vi "Translate to Array Data_BU3.vi"(8 "modified error":errorcluster, 9 "modified data":path=path "C:/Users/User/Desktop/test.csv", 10 "original error":errorcluster, 11 "original data":path=path "C:/Users/User/Desktop/aaa.csv") -> ()   [LabVIEW 2023]
uses:
  <vilib>/Utility/error.llb/DialogType.ctl
panel:
  in  "External\nRef":bool=TRUE
  out "x/y":dbl[](array[numeric])
  in  "Current Mode":u8[][](array[numeric])
  in  "Electrode number, N":u16=8
  out "number 2":i32
  out "number":i32
  in  "Only Use Last Value?":bool=TRUE
  in  "Array Mode":u16(ring) items=["Gradient + Dipole dipole", "Gradient", "Dipole Dipole", "Schlumberger"]
  in  "Insert\nBreak":bool=TRUE
  in  "Inverse\nPolarity":bool=TRUE
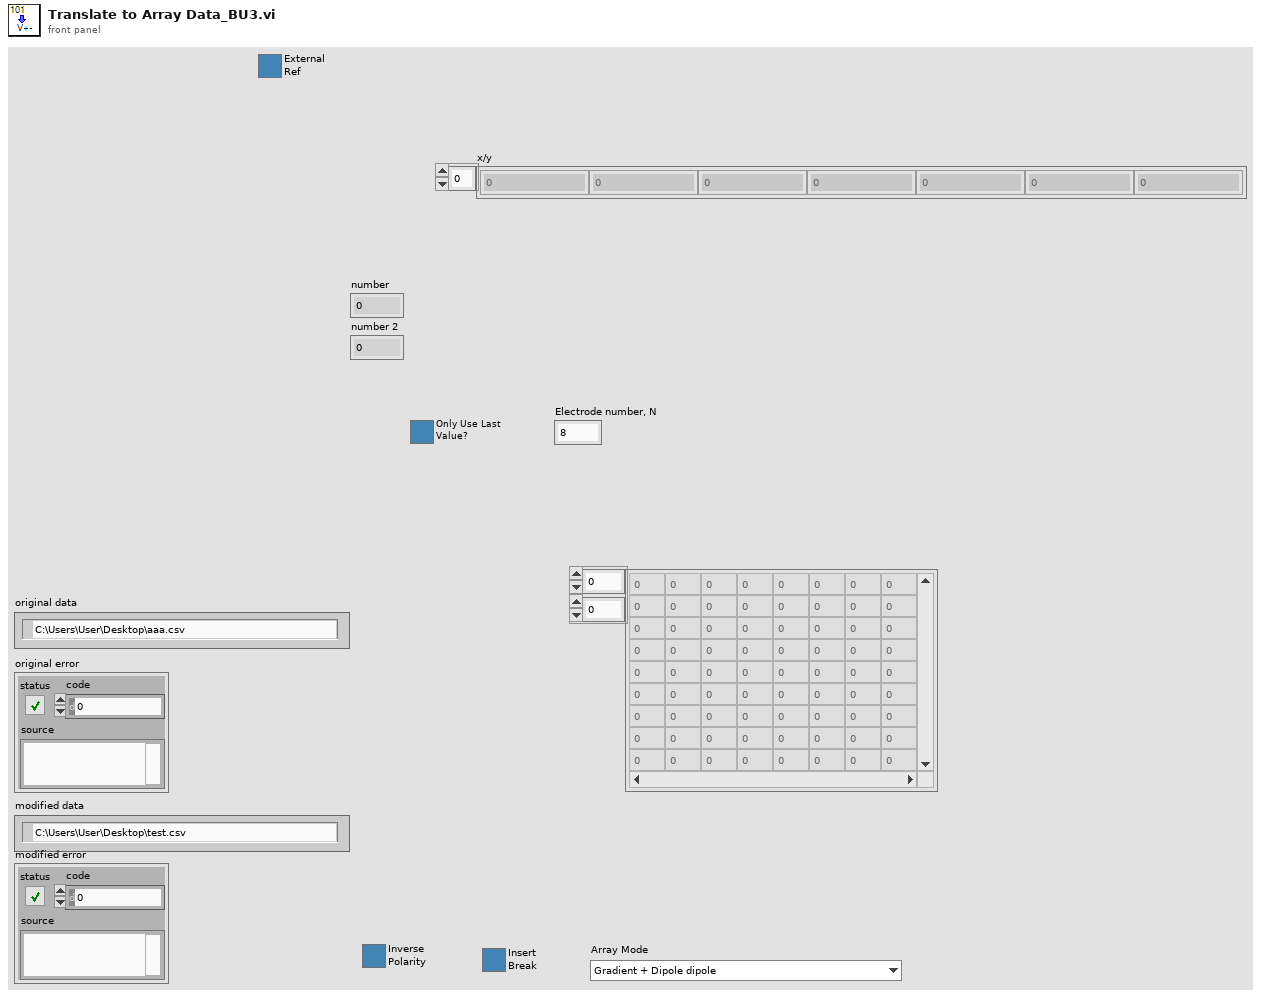
[diagram p1: front panel]
types:
  T1 = enum16{"open", "replace", "create", "open or create", "replace or create", "replace or create with confirmation"}
  T2 = typedef "DialogType.ctl" = u16
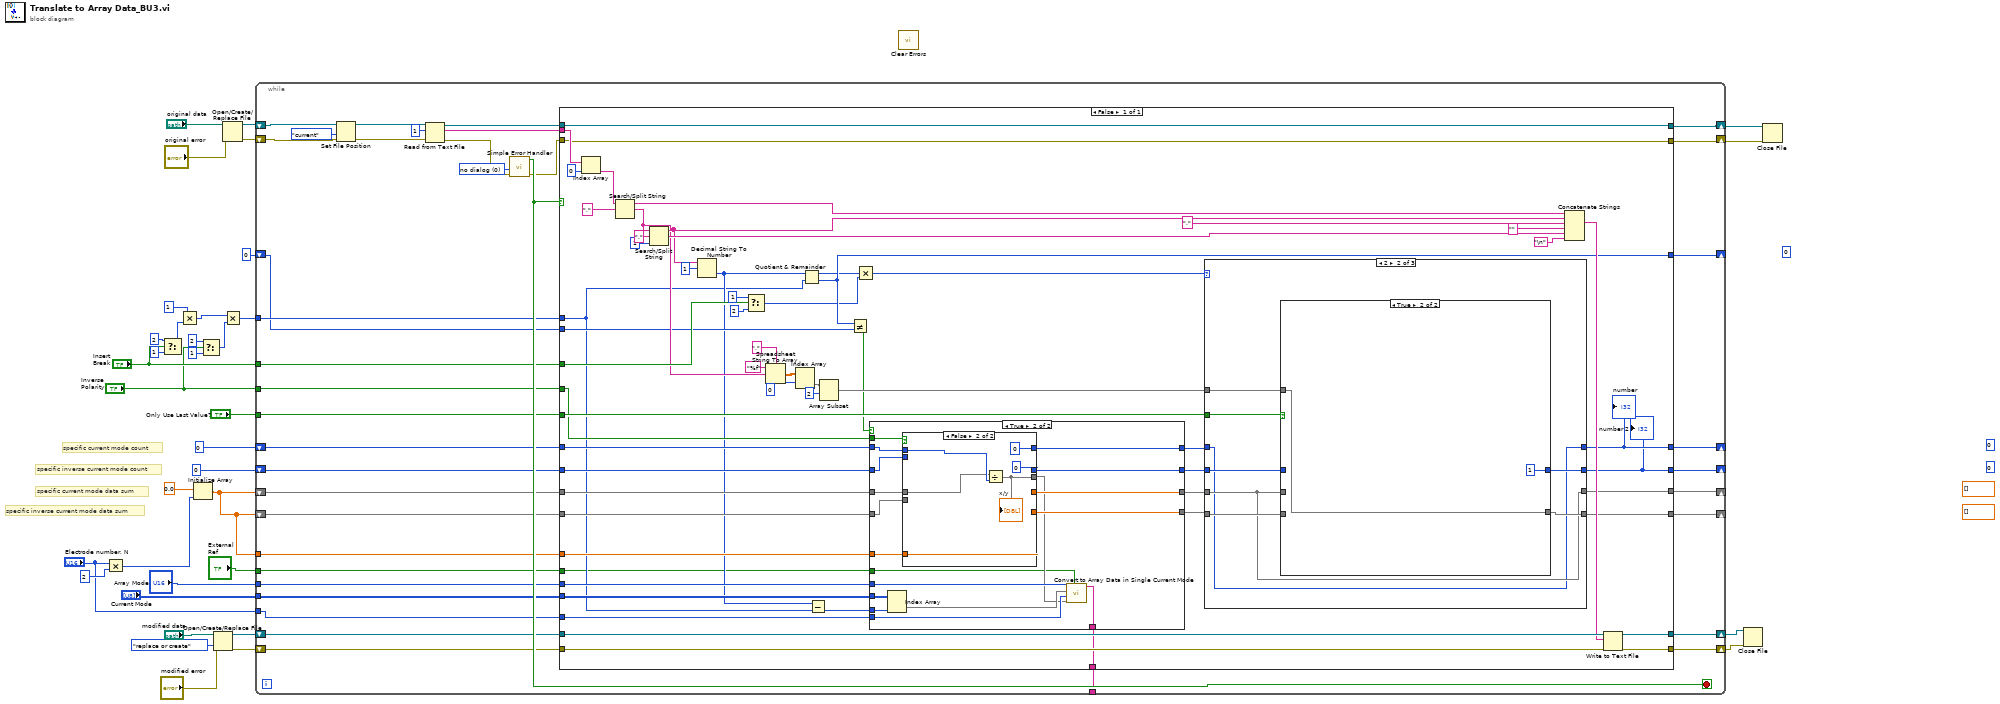
[diagram p0: block diagram]
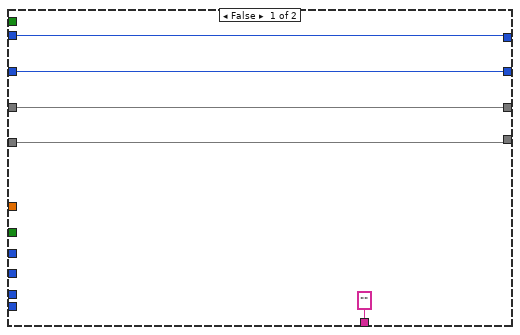
[diagram p2: hidden frame]
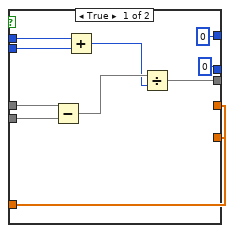
[diagram p3: hidden frame]
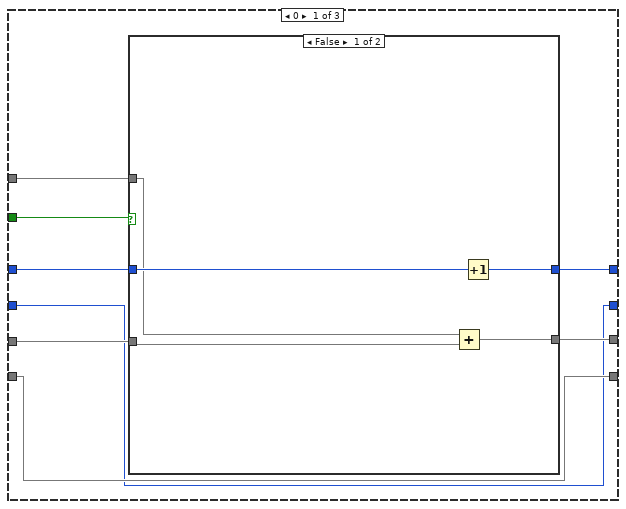
[diagram p4: hidden frame]
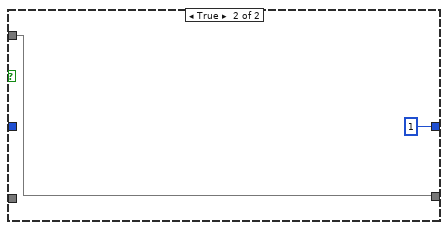
[diagram p5: hidden frame]
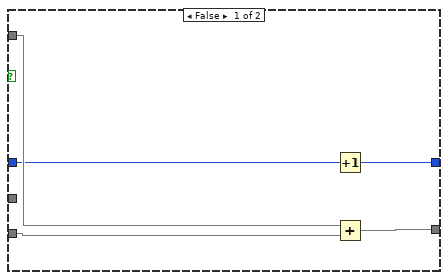
[diagram p6: hidden frame]
diagram:
  (unwired) dbl[] [] ("subarray")
  (unwired) dbl[] [] ("subarray")
  (unwired) 0 ("number")
  (unwired) 0 ("number")
  w1 = 0
  # "specific inverse current mode data sum"
  # "specific current mode data sum"
  # "specific inverse current mode count"
  # "specific current mode count"
  n1 = Multiply(x="Electrode number, N", y=u16 2) -> (x*y=w7:u16)
  n2 = Select(t=2 ("number"), s="Insert\nBreak", f=1 ("number")) -> (s? t:f=w16:i32)
  n3 = Multiply(x=1 ("number"), y=w16) -> (x*y=w10:i32)
  n4 = Initialize Array(0.0 ("element"), w7) -> (w6:dbl[])
  n5 = Select(t=2 ("number"), s="Inverse\nPolarity", f=1 ("number")) -> (s? t:f=w15:i32)
  n6 = Open/Create/Replace File(file path (use dialog)="modified data", error in="modified error", operation (0:open)=T1."replace or create") -> (refnum out=w32:refnum<file>, error out=w31:errorcluster)  [unwired: 3 in, 1 out]
  n7 = Open/Create/Replace File(file path (use dialog)="original data", error in="original error") -> (refnum out=w34:refnum<file>, error out=w35:errorcluster)  [unwired: 4 in, 1 out]
  n8 = Multiply(x=w10, y=w15) -> (x*y=w14:i32)
  n9 = while {
    shift-right: [w67] -> w25
    shift-left: w35 -> [w74]
    shift-right: [w66] -> w36
    shift-left: w34 -> [w65]
    shift-right: [w60] -> w27
    shift-left: w32 -> [w62]
    shift-right: [w59] -> w26
    shift-left: w31 -> [w61]
    tunnel: "Insert\nBreak" -> [w57]
    tunnel: "Inverse\nPolarity" -> [w56]
    tunnel: "Only Use Last Value?" -> [w55]
    tunnel: w14 -> [w54]
    shift-right: [w49] -> _
    shift-left: 0 ("number") -> [w53]
    shift-right: [w46] -> _
    shift-left: 0 ("number") -> [w52]
    shift-right: [w48] -> _
    shift-left: w6 -> [w51]
    shift-right: [w47] -> _
    shift-left: w6 -> [w50]
    shift-right: [w45] -> _
    shift-left: 0 -> [w44]
    tunnel: w6 -> [w43]
    tunnel: "Current Mode" -> [w41]
    tunnel: "Array Mode" -> [w42]
    tunnel: "Electrode number, N" -> [w40]
    tunnel: "External\nRef" -> [w39]
    tunnel: [w38] -> _
    stop <- w71 stop-if-true
    w72 = T2 0 items=["no dialog", "OK message", "continue or stop message", "OK message + warnings", "continue/stop + warnings"] ("type of dialog (OK msg:1)")
    n10 = Set File Position(refnum=w65, from (0:start)=enum16{"start", "end", "current"}."current", error in=w74) -> (refnum out=w64:refnum<file>, error out=w63:errorcluster)  [unwired: 1 in]
    n11 = Read from Text File(file (use dialog)=w64, count=1, error in=w63) -> (refnum out=w69:refnum<file>, text=w70:string[], error out=w68:errorcluster)  [unwired: 1 in, 1 out]
    n12 = call <vilib>:"Simple Error Handler.vi"("type of dialog (OK msg:1)"=w72, "error in (no error)"=w68) -> ("error?"=w71:bool, "error out"=w58:errorcluster)  [unwired: 3 in, 3 out]
    n13 = case shown="False" w71 {
      tunnel: w70 -> [w129]
      tunnel: w69 -> [w126]
      tunnel: w58 -> [w125]
      tunnel: [w126] -> w66
      tunnel: [w125] -> w67
      tunnel: w62 -> [w124]
      tunnel: w61 -> [w123]
      tunnel: [w122] -> w60
      tunnel: [w121] -> w59
      tunnel: w57 -> [w115]
      tunnel: w56 -> [w93]
      tunnel: w55 -> [w113]
      tunnel: w54 -> [w79]
      tunnel: w53 -> [w97]
      tunnel: w52 -> [w96]
      tunnel: w51 -> [w95]
      tunnel: w50 -> [w94]
      tunnel: [w103] -> w49
      tunnel: [w102] -> w48
      tunnel: [w101] -> w47
      tunnel: [w100] -> w46
      tunnel: [w98] -> w45
      tunnel: w44 -> [w99]
      tunnel: w43 -> [w87]
      tunnel: w42 -> [w83]
      tunnel: w41 -> [w82]
      tunnel: w40 -> [w78]
      tunnel: w39 -> [w77]
      tunnel: [w76] -> w38
      frame False {
        n14 = Index Array(array=w129, index=0) -> (element=w127:string)
        n15 = Search/Split String(string=w127, search string/char (-)=",") -> (substring before match=w135:string, match + rest of string=w109:string)  [unwired: 1 in, 1 out]
        n16 = Search/Split String(string=w109, search string/char (-)=",", offset (0)=1) -> (substring before match=w110:string, match + rest of string=w118:string)  [unwired: 1 out]
        n17 = Decimal String To Number(string=w110, offset=1) -> (number=w80:i32)  [unwired: 1 in, 1 out]
        n18 = Select(t=1, s=w115, f=2 ("y")) -> (s? t:f=w86:i32)
        n19 = Spreadsheet String To Array(delimiter (Tab)=",", format string="%f", spreadsheet string=w109) -> (array=w108:dbl[][])  [unwired: 1 in]
        n20 = Index Array(array=w108, index (row)=0) -> (element=w106:dbl[])  [unwired: 1 in]
        n21 = Quotient & Remainder(x=w80, y=w79) -> (x-y*floor(x/y)=w85:i32, floor(x/y)=w98:i32)
        n22 = Subtract(x=w80, y=w79) -> (x-y=w81:i32)
        n23 = Array Subset(array=w106, index=2) -> (w104:dbl[])  [unwired: 1 in]
        n24 = Not Equal?(x=w98, y=w99) -> (x != y?=w88:bool)
        n25 = Multiply(x=w85, y=w86) -> (x*y=w84:i32)
        n26 = case shown="True" w88 {
          tunnel: w97 -> [w140 w155]
          tunnel: w96 -> [w139 w154]
          tunnel: w95 -> [w138 w157]
          tunnel: w94 -> [w137 w156]
          tunnel: w93 -> [_ w158]
          tunnel: [w140 w153] -> w92
          tunnel: [w139 w152] -> w91
          tunnel: [w138 w151] -> w90
          tunnel: [w137 w150] -> w89
          tunnel: w87 -> [_ w149]
          tunnel: w83 -> [_ w145]
          tunnel: w82 -> [_ w148]
          tunnel: w81 -> [_ w147]
          tunnel: w78 -> [_ w144]
          tunnel: w77 -> [_ w142]
          tunnel: ["" ("String") w141] -> w76
          frame False {
          }
          frame True {
            n27 = Index Array(array=w148, index (col)=w147) -> (element=w146:u8[])  [unwired: 1 in]
            n28 = case shown="False" w158 {
              tunnel: w157 -> [w168 w171]
              tunnel: w156 -> [w167 _]
              tunnel: w155 -> [w166 w172]
              tunnel: w154 -> [w165 _]
              tunnel: [0 ("number") 0 ("number")] -> w153
              tunnel: [0 ("number") 0 ("number")] -> w152
              tunnel: [w160 w170] -> w151
              tunnel: [w160 w170] -> w150
              tunnel: w149 -> [w160 w170]
              tunnel: [w159 w169] -> w143
              frame True {
                n29 = Subtract(x=w168, y=w167) -> (x-y=w164:dbl[])
                n30 = Add(x=w166, y=w165) -> (x+y=w163:i32)
                n31 = Divide(x=w164, y=w163) -> (x/y=w159:dbl[])
              }
              frame False {
                n32 = Divide(x=w171, y=w172) -> (x/y=w169:dbl[])
                "x/y" <- w169
              }
            }
            n33 = call "Convert to Array Data in Single Current Mode.vi"("External\nRef"=w142, "data"=w143, "Electrode number, N"=w144, "Current Mode"=w146, "Array Mode"=w145) -> ("String"=w141:string)  [unwired: 6 in]
          }
        }
        n34 = case shown="2" w84 {
          tunnel: w113 -> [w182 w197 _]
          tunnel: w104 -> [w178 w196 _]
          tunnel: w92 -> [w181 w190 w208]
          tunnel: w91 -> [w175 w193 w207]
          tunnel: w90 -> [w180 w191 w206]
          tunnel: w89 -> [w176 w195 w205]
          tunnel: [w179 w190 w208] -> w103
          tunnel: [w177 w191 w206] -> w102
          tunnel: [w176 w194 w205] -> w101
          tunnel: [w175 w192 w207] -> w100
          frame 0 {
            n35 = case shown="False" w182 {
              tunnel: w181 -> [w187 _]
              tunnel: w180 -> [w184 _]
              tunnel: [w186 1 ("number")] -> w179
              tunnel: w178 -> [w183 w188]
              tunnel: [w185 w188] -> w177
              frame False {
                n36 = Add(x=w183, y=w184) -> (x+y=w185:dbl[])
                n37 = Increment(x=w187) -> (x+1=w186:i32)
              }
              frame True {
              }
            }
          }
          frame 2 {
            n38 = case shown="True" w197 {
              tunnel: w191 -> [_ _]
              tunnel: w196 -> [w201 w204]
              tunnel: [w202 w204] -> w194
              tunnel: w195 -> [w200 _]
              tunnel: w193 -> [w199 _]
              tunnel: [w198 1 ("number")] -> w192
              frame False {
                n39 = Increment(x=w199) -> (x+1=w198:i32)
                n40 = Add(x=w201, y=w200) -> (x+y=w202:dbl[])
              }
              frame True {
              }
            }
          }
          frame 1, 3, Default {
          }
        }
        "number" <- w103
        "number 2" <- w100
        n41 = Concatenate Strings(w135, w110, "," ("string"), "" ("string"), w118, "\n") -> (w120:string)
        n42 = Write to Text File(file (use dialog)=w124, text=w120, error in=w123) -> (refnum out=w122:refnum<file>, error out=w121:errorcluster)  [unwired: 1 in, 1 out]
      }
    }
  }
  n43 = call <vilib>:"Clear Errors.vi"() -> ()  [unwired: 6 in, 2 out]
  n44 = Close File(refnum=w27, error in=w26) -> ()  [unwired: 2 out]
  n45 = Close File(refnum=w36, error in=w25) -> ()  [unwired: 2 out]
